vi "Create Observer.vi"(8 "error in (no error)":errorcluster, 11 "Actor in":refnum<class "Actor.lvclass">) -> (0 "error out":errorcluster, 2 "Actor":refnum<event-registration>, 3 "Actor out":refnum<class "Actor.lvclass">)   [LabVIEW 2015, in "Actor.lvclass"]
doc: "Registers a User Event from the Request Channel.\n\nThis is used to create the mechanism that handles the requests (from outside this Actor) into this Actor."
uses:
  Actor.lvclass
  Messaging/Message/Message.lvclass
  Actor.lvclass/Actor.ctl
  Messaging/Messenger/Messenger.lvclass
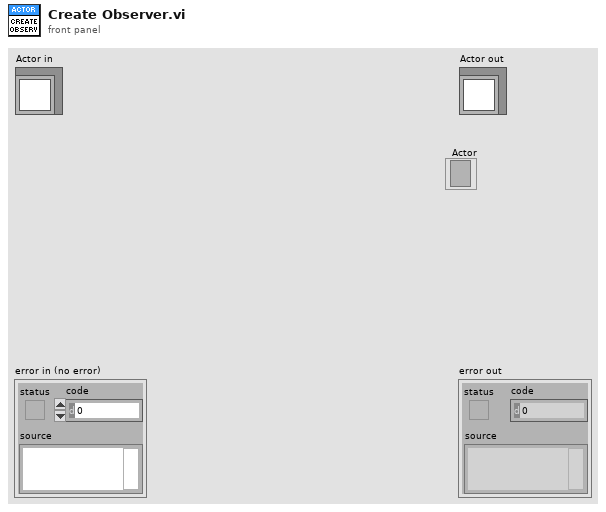
[diagram p1: front panel]
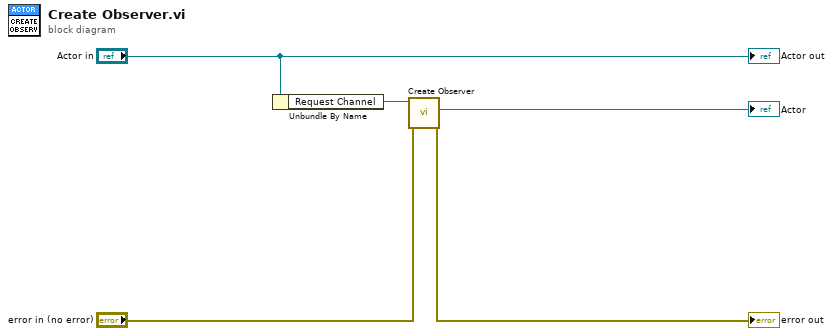
[diagram p0: block diagram]
diagram:
  n1 = Unbundle By Name("Actor in") -> ("Request Channel"=w1:refnum<class "Messenger.lvclass">)
  n2 = call "Create Observer.vi"("error in (no error)"="error in (no error)", "Messenger in"=w1) -> ("error out"=→"error out":errorcluster, "Observer"=→"Actor":refnum<event-registration>)  [unwired: 7 in, 1 out]
  "Actor out" <- "Actor in"
